vi "Tablet dummy xbox Main.vi"() -> ()   [LabVIEW 2009]
uses:
  Remote Control/Control Message.ctl
  Remote Control/Motor Command.ctl
  UDP Lib/UDP Network Location.ctl
panel:
  in  "RC/!AT":bool
  in  "Control Message":T1
  in  "Speed":i32=1
  in  "Turn":i32=1
  in  "STOP":bool
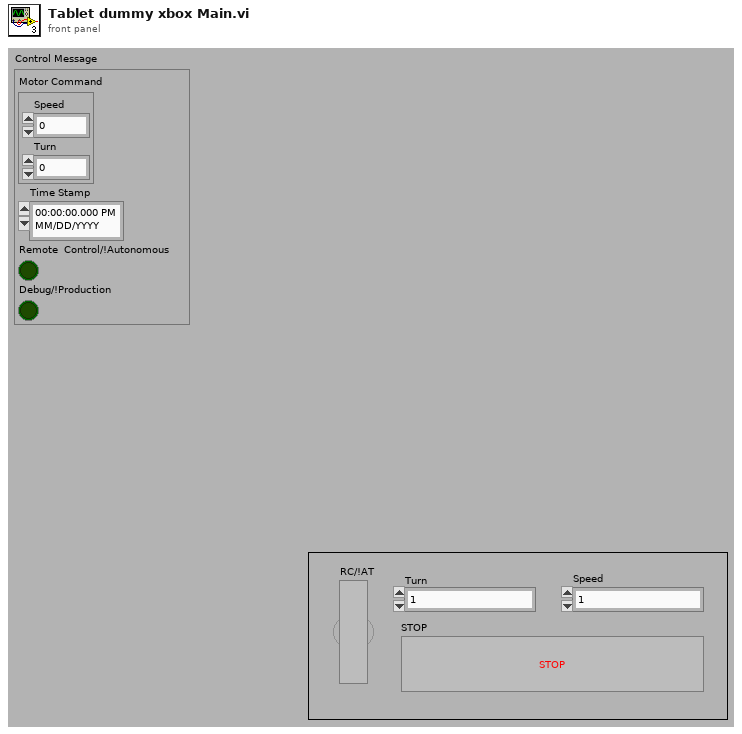
[diagram p1: front panel]
types:
  T1 = typedef "Control Message.ctl" = cluster{"Motor Command":T2, "Time Stamp":timestamp, "Remote  Control/!Autonomous":bool, "Debug/!Production":bool}
  T2 = typedef "Motor Command.ctl" = cluster{"Speed":i16, "Turn":i16}
  T3 = typedef "UDP Base.ctl" = cluster{"UDP Session":refnum<k16>, "UDP Socket Params":T4}
  T4 = typedef "UDP Socket Params.ctl" = cluster{"Local Port":u16, "Read Timeout":i32, "Write Timeout":i32}
  T5 = typedef "UDP Network Location.ctl" = cluster{"IP Address":string, "Port":u16}
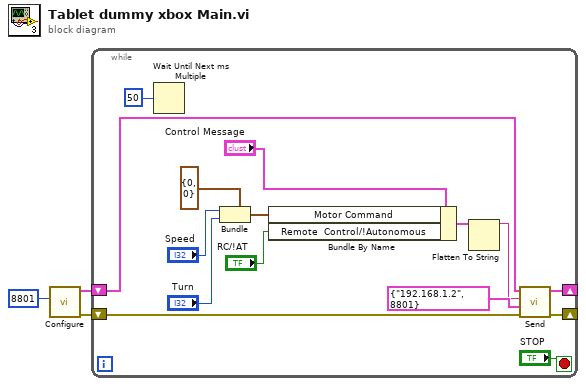
[diagram p0: block diagram]
diagram:
  n1 = call "Configure.vi"("Local Port"=u16 8801) -> ("error out"=w2:errorcluster, "UDP Base out"=w1:T3)  [unwired: 9 in]
  n2 = while {
    shift-right: [w13] -> _
    shift-left: w1 -> [w15]
    shift-right: [w12] -> _
    shift-left: w2 -> [w17]
    stop <- "STOP" stop-if-true
    n3 = Wait Until Next ms Multiple(millisecond multiple=u32 50) -> ()  [unwired: 1 out]
    n4 = Bundle(cluster=T2 {"Speed"=0, "Turn"=0} ("Motor Command"), "Speed"="Speed", "Turn"="Turn") -> (w8:T2)
    n5 = Bundle By Name(cluster="Control Message", "Motor Command"=w8, "Remote  Control/!Autonomous"="RC/!AT") -> (w4:T1)
    n6 = Flatten To String(anything=w4) -> (data string=w14:string)  [unwired: 3 in, 2 out]
    n7 = call "Send.vi"("error in (no error)"=w17, "Destination Location"=T5 {"IP Address"="192.168.1.2", "Port"=8801}, "Send Data"=w14, "UDP Base in"=w15) -> ("error out"=w12:errorcluster, "UDP Base out"=w13:T3)  [unwired: 5 in, 1 out]
  }
